vi "Actor Core.vi"(8 "error in":errorcluster, 11 "Caller in":refnum<class "Caller.lvclass">) -> (0 "error out":errorcluster, 3 "Actor out":refnum<class "Actor.lvclass">)   [LabVIEW 2020, in "Caller.lvlib" / "Caller.lvclass"]
doc: "(<B>Filename</B>: Actor Framework.lvlib:Actor.lvclass:Actor Core.vi)\n\nReceives messages to the actor, reacts to them, and initiates any error handling that may shut the actor down.\n\nDescendant classes may override this VI to append parallel tasks for the actor to complete while it handles messages. Overrides use the Call Parent Class Method node."
uses:
  Caller.lvclass
  <vilib>/ActorFramework/Actor/Actor.lvclass
  Caller.lvclass/Caller.ctl
  Caller Messages/UpdateMessage Msg/UpdateMessage Msg.lvclass/UpdateMessage Msg.ctl
  <vilib>/ActorFramework/Message Enqueuer/Message Enqueuer.lvclass/Message Enqueuer.ctl
  _ctrl/ctrl_ref.ctl
  Caller Messages/InitRef Msg/InitRef Msg.lvclass/InitRef Msg.ctl
  <vilib>/ActorFramework/Message Enqueuer/Enqueue.vi
  Caller Messages/UpdateMessage Msg/UpdateMessage Msg.lvclass
  C:/Program Files/National Instruments/LabVIEW 2020/vi.lib/ActorFramework/Message/Message.lvclass
  Caller Messages/ErrorState Msg/ErrorState Msg.lvclass
  <vilib>/ActorFramework/Stop Msg/Stop Msg.lvclass
  Caller Messages/InitRef Msg/InitRef Msg.lvclass
  <vilib>/ActorFramework/Message Priority Queue/Priority Enqueue.vi
panel:
  out "Message_cpt":u8
  in  "Btn_Error":bool
  in  "Btn_Launch":bool
  in  "Message":string
  out "Display":string
  in  "Btn_ Send":bool
  # "Caller"
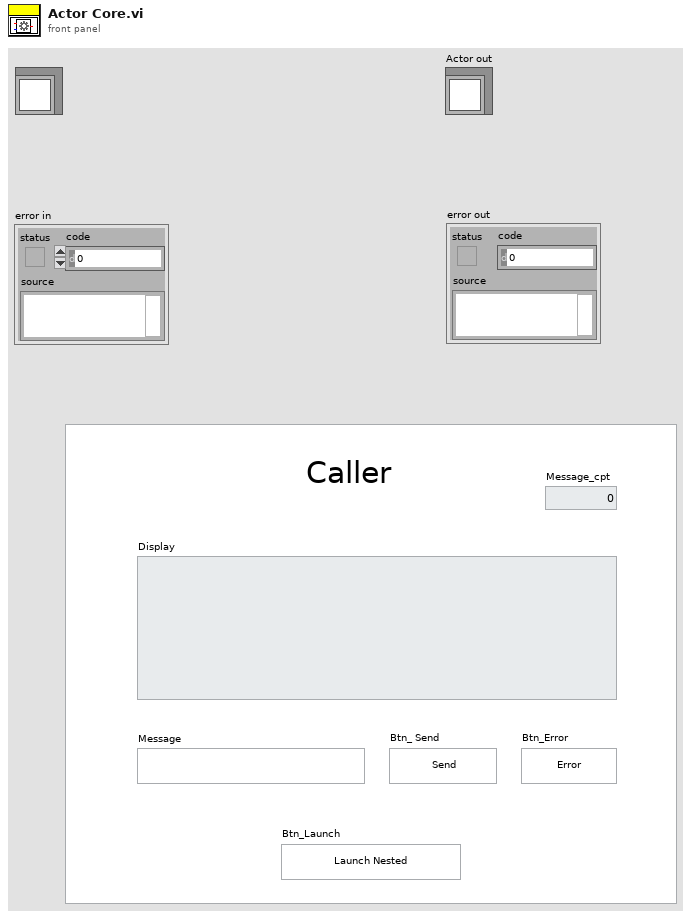
[diagram p1: front panel]
types:
  T1 = typedef "ctrl_ref.ctl" = cluster{"Message_cpt":refnum<vi>}
  T2 = cluster{"Quit":refnum<user-event>, "UpdateDisplay":refnum<user-event>, "DisplayCompteur":refnum<user-event>}
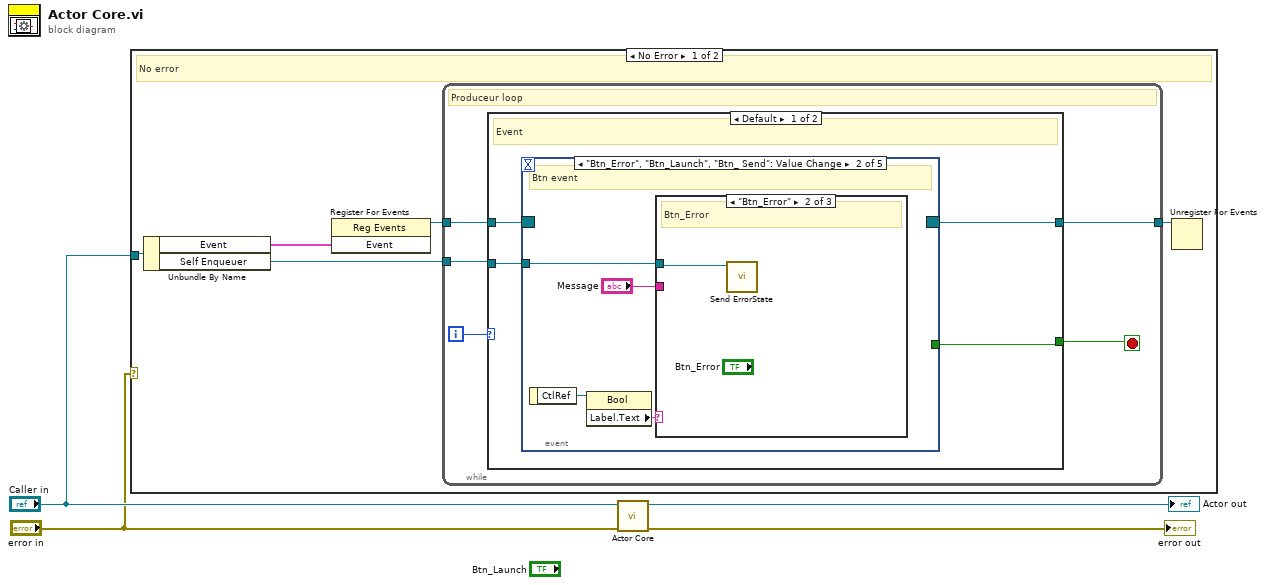
[diagram p0: block diagram]
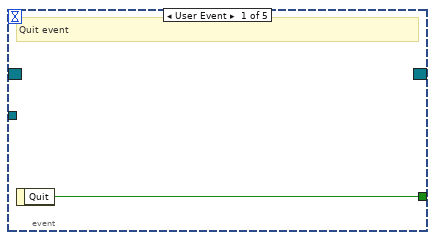
[diagram p2: hidden frame]
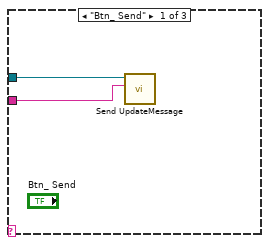
[diagram p3: hidden frame]
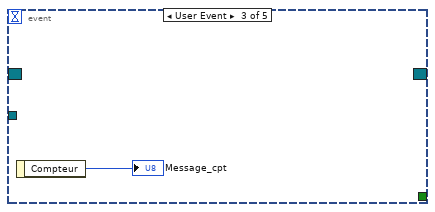
[diagram p5: hidden frame]
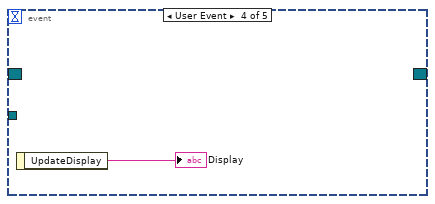
[diagram p6: hidden frame]
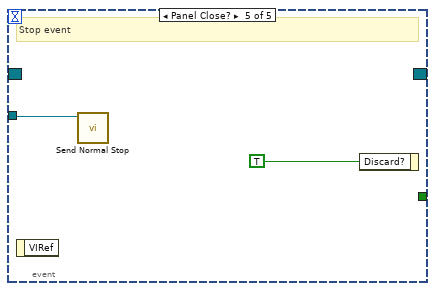
[diagram p7: hidden frame]
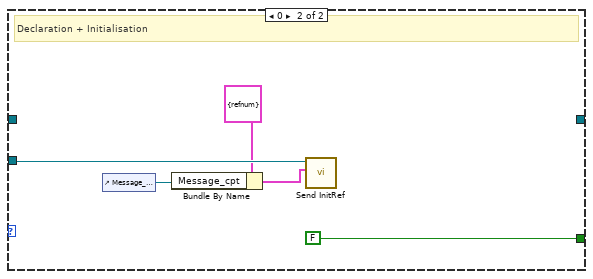
[diagram p8: hidden frame]
diagram:
  n1 = case shown="No Error" "error in" {
    tunnel: "Caller in" -> [w7 _]
    frame No Error {
      # "No error"
      n2 = Unbundle By Name(w7) -> ("Event"=w5:T2, "Self Enqueuer"=w8:refnum<class "Message Enqueuer.lvclass">)
      n3 = register-events(w5) -> (reference out=w6:refnum<event-registration>)  [unwired: 2 in, 1 out]
      n4 = while {
        tunnel: [w12] -> w9
        tunnel: w8 -> [w11]
        tunnel: w6 -> [w10]
        i -> [w14]
        stop <- w13 stop-if-true
        # "Produceur loop"
        n5 = case shown="Default" w14 {
          tunnel: w11 -> [w16 w34]
          tunnel: [w17 FALSE] -> w13
          tunnel: [w18 _] -> w12
          tunnel: w10 -> [w15 _]
          frame Default {
            # "Event"
            n6 = event shown="[1] \"Btn_Error\", \"Btn_Launch\", \"Btn_ Send\": Value Change" {
              selector: w15 -> [_ _ _ _ _]
              dyn-events: [_ _ _ _ _] -> w18
              timeout: _ -> [_ _ _ _ _]
              tunnel: [w19 _ _ _ _] -> w17
              tunnel: w16 -> [_ w21 _ _ w29]
              event User Event {
                # "Quit event"
                n7 = event-data() -> ("Quit"=w19:bool)  [unwired: 1 in]
              }
              event "Btn_Error", "Btn_Launch", "Btn_ Send": Value Change {
                # "Btn event"
                n8 = event-data() -> ("CtlRef"=w23:refnum<vi>)  [unwired: 1 in]
                n9 = property class="Bool"(reference=w23) -> ("Label.Text"=w22:string)  [unwired: 1 in, 2 out]
                n10 = case shown="\"Btn_Error\"" w22 {
                  tunnel: w21 -> [w25 w26 _]
                  tunnel: "Message" -> [w24 _ _]
                  frame "Btn_ Send" {
                    n11 = call "Send UpdateMessage.vi"("Message"=w24, "Message Enqueuer"=w25) -> ()  [unwired: 8 in, 2 out]
                  }
                  frame "Btn_Error" {
                    # "Btn_Error"
                    n12 = call "Send ErrorState.vi"("Message Enqueuer"=w26) -> ()  [unwired: 9 in, 2 out]
                  }
                  frame Default {
                    # "Do nothing"
                  }
                }
              }
              event User Event {
                n13 = event-data() -> ("Compteur"=→"Message_cpt":u8)  [unwired: 1 in]
              }
              event User Event {
                n14 = event-data() -> ("UpdateDisplay"=→"Display":string)  [unwired: 1 in]
              }
              event Panel Close? {
                # "Stop event"
                n15 = event-data() -> ()  [unwired: 1 in, 1 out]
                n16 = call <vilib>:"Send Normal Stop.vi"("Message Enqueuer"=w29) -> ()  [unwired: 10 in, 1 out]
                n17 = event-data("Discard?"=TRUE) -> ()  [unwired: 1 in, 1 out]
              }
            }
          }
          frame 0 {
            # "Declaration + Initialisation"
            n18 = control-ref of="Message_cpt"() -> (w31:refnum<vi>)
            n19 = Bundle By Name(cluster=T1 {"Message_cpt"=refnum} ("Ref"), "Message_cpt"=w31) -> (w32:T1)
            n20 = call "Send InitRef.vi"("Ref"=w32, "Message Enqueuer"=w34) -> ()  [unwired: 8 in, 2 out]
          }
        }
      }
      n21 = Unregister For Events(event registration refnum=w9) -> ()  [unwired: 1 in, 1 out]
    }
    frame Error {
    }
  }
  n22 = call-parent "Actor Core.vi"("error in"="error in", "Actor in"="Caller in") -> ("error out"=→"error out":errorcluster, "Actor out"=→"Actor out":refnum<class "Actor.lvclass">)  [unwired: 8 in]
